vi "Configure.vi"(8 "error in (no error)":errorcluster, 10 "new cameras":T6[](array[typedef]), 11 "config":T1={"active cameras"=[], "poll interval (sec)"=1.0}) -> (0 "error out":errorcluster, 1 "error cameras":T2[](array[typedef]), 2 "new cameras":T2[](array[typedef]), 3 "config out":T1={"active cameras"=[], "poll interval (sec)"=1.0}, 4 "error text":string[](array[string]))   [LabVIEW 2017, in "IrAcquisition.lvlib"]
uses:
  <vilib>/addons/InsightCM/Devices/Shared/Ir/IrAcquisition/IrAcquisition.lvlib
  <vilib>/addons/InsightCM/Devices/Shared/Ir/IrAcquisition/controls/config.ctl
  <vilib>/addons/InsightCM/Devices/Shared/Ir/IrAcquisition/controls/camera.ctl
  <vilib>/userdefined/High Color/IMAQdx.ctl
  <vilib>/vision/Image Controls.llb/IMAQ Image.ctl
  <vilib>/addons/PointValueMap/controls/PointMap.ctl
  <vilib>/addons/InsightCM/Devices/Shared/Ir/IrManageCameras/controls/camera.ctl
  <vilib>/addons/PointValueMap/PointValueMap.lvlib
  <vilib>/addons/InsightCM/Utilities/GlobalConfiguration/GlobalConfiguration.lvlib
  <vilib>/addons/InsightCM/Utilities/DeviceModelHelpers/DeviceModelHelpers.lvlib
  <vilib>/addons/InsightCM/Devices/Shared/Ir/IrManageCameras/IrManageCameras.lvlib
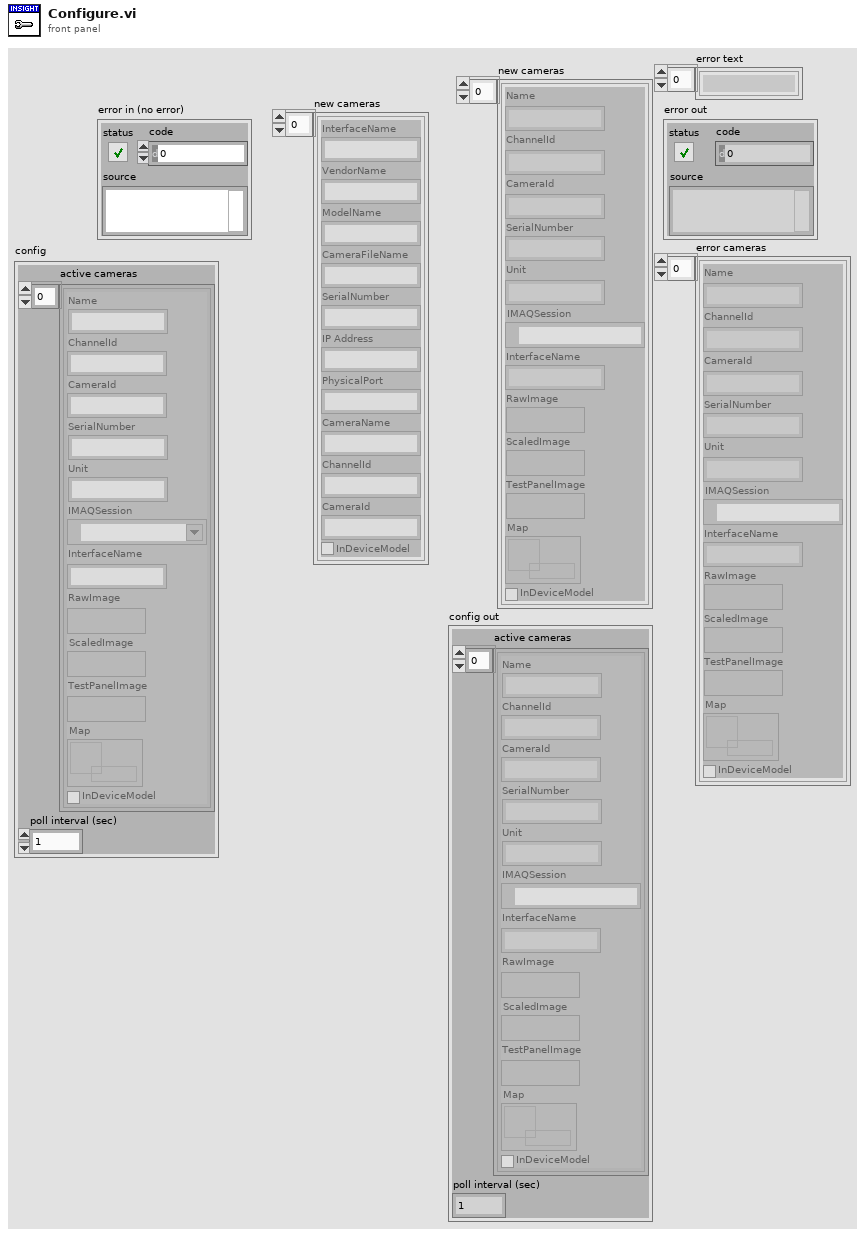
[diagram p1: front panel]
types:
  T1 = typedef "IrAcquisition.lvlib/config.ctl" = cluster{"active cameras":T2[], "poll interval (sec)":dbl}
  T2 = typedef "IrAcquisition.lvlib/camera.ctl" = cluster{"Name":string, "ChannelId":string, "CameraId":string, "SerialNumber":string, "Unit":string, "IMAQSession":T3, "InterfaceName":string, "RawImage":T4, "ScaledImage":T4, "TestPanelImage":T4, "Map":T5, "InDeviceModel":bool}
  T3 = typedef "IMAQdx.ctl" = refnum<k21>
  T4 = typedef "IMAQ Image.ctl" = refnum<image>
  T5 = typedef "PointValueMap.lvlib/PointMap.ctl" = refnum<data-value>
  T6 = typedef "IrManageCameras.lvlib/camera.ctl" = cluster{"InterfaceName":string, "VendorName":string, "ModelName":string, "CameraFileName":string, "SerialNumber":string, "IP Address":string, "PhysicalPort":string, "CameraName":string, "ChannelId":string, "CameraId":string, "InDeviceModel":bool}
  T7 = typedef "Camera.ctl" = cluster{"Id":string, "Name":string, "Properties":T8[], "Triggers":T9[]}
  T8 = typedef "KeyValuePair.ctl" = cluster{"Key":string, "Value":string}
  T9 = typedef "Trigger.ctl" = cluster{"Type":string, "Expression":string, "Conditions":T10[]}
  T10 = typedef "Condition.ctl" = cluster{"Source":string, "Type":string, "Operator":string, "CompareTo":string, "DwellSeconds":dbl}
  T11 = typedef "IrAcquisition.lvlib/IRCameraSettings.ctl" = cluster{"emissitivity":dbl, "reflected temperature":dbl, "window transmission":dbl, "window temperature":dbl, "atmospheric transmission":dbl, "atmospheric temperature":dbl}
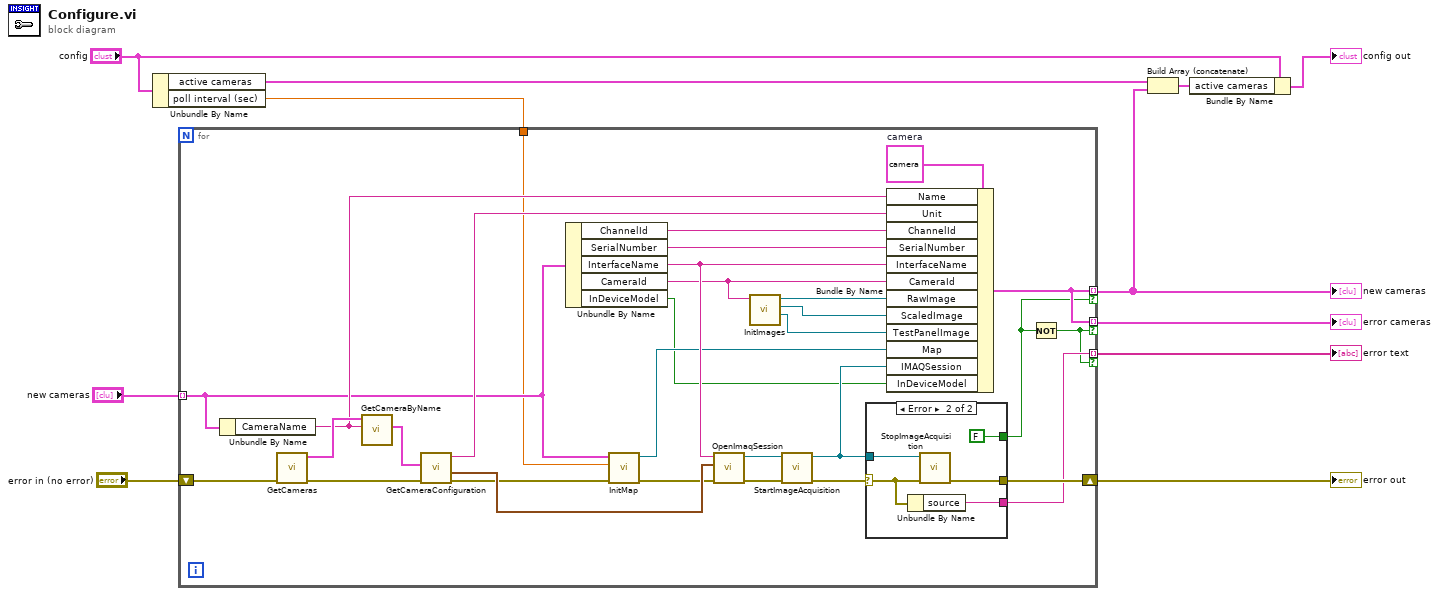
[diagram p0: block diagram]
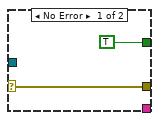
[diagram p2: hidden frame]
diagram:
  n1 = Unbundle By Name("config") -> ("active cameras"=w5:T2[], "poll interval (sec)"=w6:dbl)
  n2 = for {
    shift-right: [w41] -> w11
    shift-left: "error in (no error)" -> [w40]
    tunnel: "new cameras" -> [w18] mode=indexing
    tunnel: [w17] -> w4 mode=indexing if=w16
    tunnel: [w17] -> w8 mode=indexing if=w12
    tunnel: w6 -> [w15]
    tunnel: [w13] -> w1 mode=indexing if=w12
    w33 = T2 {"Name"="", "ChannelId"="", "CameraId"="", "SerialNumber"="", "Unit"="", "IMAQSession"="", "InterfaceName"="", "RawImage"=refnum, "ScaledImage"=refnum, "TestPanelImage"=refnum, "Map"=refnum, "InDeviceModel"=FALSE}  # camera
    n3 = Unbundle By Name(w18) -> ("CameraName"=w19:string)
    n4 = call <vilib>:"GetCameras.vi"("error in (no error)"=w40) -> ("error out"=w39:errorcluster, "cameras"=w38:T7[])  [unwired: 8 in, 1 out]
    n5 = call <vilib>:"GetCameraByName.vi"("name"=w19, "cameras in"=w38) -> ("camera"=w37:T7)  [unwired: 7 in, 2 out]
    n6 = call <vilib>:"GetCameraConfiguration.vi"("error in (no error)"=w39, "camera"=w37) -> ("error out"=w25:errorcluster, "camera settings"=w32:T11, "units"=w26:string)  [unwired: 7 in]
    n7 = Unbundle By Name(w18) -> ("ChannelId"=w27:string, "SerialNumber"=w30:string, "InterfaceName"=w34:string, "CameraId"=w20:string, "InDeviceModel"=w14:bool)
    n8 = call <vilib>:"InitMap.vi"("error in (no error)"=w25, "ImagePoll"=w15, "Camera Info"=w18) -> ("error out"=w24:errorcluster, "map out"=w28:T5)  [unwired: 7 in]
    n9 = call <vilib>:"OpenImaqSession.vi"("error in (no error)"=w24, "camera settings"=w32, "interface name"=w34) -> ("error out"=w23:errorcluster, "imaq session"=w29:T3)  [unwired: 7 in]
    n10 = call <vilib>:"InitImages.vi"("camera id"=w20) -> ("test panel image"=w35:T4, "scaled image"=w36:T4, "raw image"=w21:T4)  [unwired: 8 in]
    n11 = call <vilib>:"StartImageAcquisition.vi"("error in (no error)"=w23, "session in"=w29) -> ("error out"=w31:errorcluster, "session out"=w22:T3)  [unwired: 8 in]
    n12 = case shown="Error" w31 {
      selector: w31 -> [w43 w45]
      tunnel: w22 -> [_ w48]
      tunnel: [w43 w47] -> w41
      tunnel: [TRUE FALSE] -> w16
      tunnel: [_ w44] -> w13
      frame No Error {
      }
      frame Error {
        n13 = Unbundle By Name(w45) -> ("source"=w44:string)
        n14 = call <vilib>:"StopImageAcquisition.vi"("error in (no error)"=w45, "session in"=w48) -> ("error out"=w47:errorcluster)  [unwired: 9 in]
      }
    }
    n15 = Bundle By Name(cluster=w33, "Name"=w19, "Unit"=w26, "ChannelId"=w27, "SerialNumber"=w30, "InterfaceName"=w34, "CameraId"=w20, "RawImage"=w21, "ScaledImage"=w36, "TestPanelImage"=w35, "Map"=w28, "IMAQSession"=w22, "InDeviceModel"=w14) -> (w17:T2)
    n16 = Not(x=w16) -> (.not. x?=w12:bool)
  }
  "error out" <- w11
  "new cameras" <- w4
  "error cameras" <- w8
  "error text" <- w1
  n17 = Build Array (concatenate)(w5, w4) -> (w3:T2[])
  n18 = Bundle By Name(cluster="config", "active cameras"=w3) -> (→"config out":T1)
